vi "SelectData.vi"(8 "error in (no error)":errorcluster, 10 "Select Conditions Criteria":T1, 11 "object in":refnum<class "TableLogger_SQLite_Actor.lvclass">) -> (0 "error out":errorcluster, 2 "Data Clusters":variant[](array[variant]), 3 "object out":refnum<class "TableLogger_SQLite_Actor.lvclass">)   [LabVIEW 2014, in "TableLogger_SQLite_Actor.lvlib" / "TableLogger_SQLite_Actor.lvclass"]
uses:
  TableLogger_SQLite_Actor.lvclass
  TableLogger_Actor/SelectConditionCriteria.ctl
  SelectConditions.ctl
  TableLogger_SQLite_Actor.lvclass/TableLogger_SQLite_Actor.ctl
  <vilib>/drjdpowell/SQLite Library/SQL Connection/Execute SQL.vi
  <vilib>/drjdpowell/SQLite Library/SQLite.lvlib
  <vilib>/drjdpowell/SQLite Library/SQL Connection/Connection.lvclass
  TableLogger_Actor/TableLogger_Actor/TableLogger_Actor.lvclass
  TableLogger_Actor/TableLogger_Actor.lvlib
panel:
  # "Connector Pane"
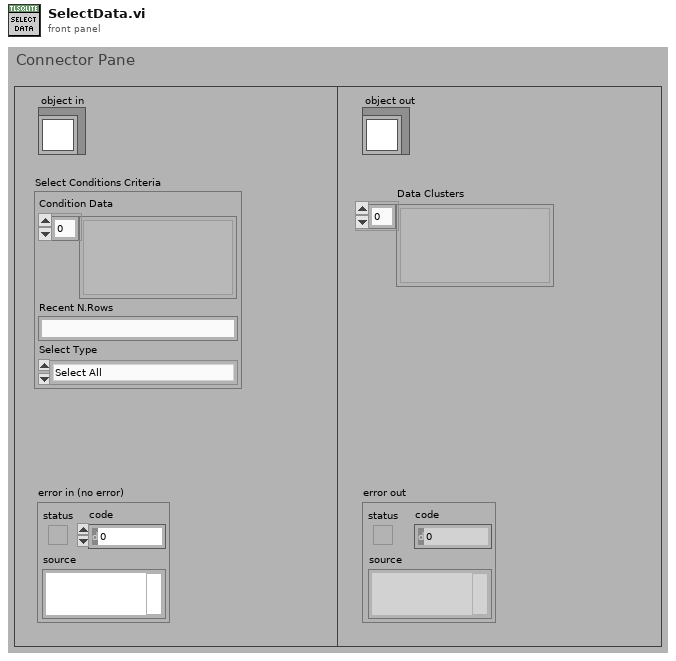
[diagram p1: front panel]
types:
  T1 = typedef "TableLogger_Actor.lvlib/SelectConditionCriteria.ctl" = cluster{"Condition Data":variant[], "Recent N.Rows":string, "Select Type":T2}
  T2 = typedef "TableLogger_Actor.lvlib/SelectConditions.ctl" = enum16{"Select All", "Select with AND Operator", "Select Most Recent Rows", "Select with OR Operator", "Select with BETWEEN Operator"}
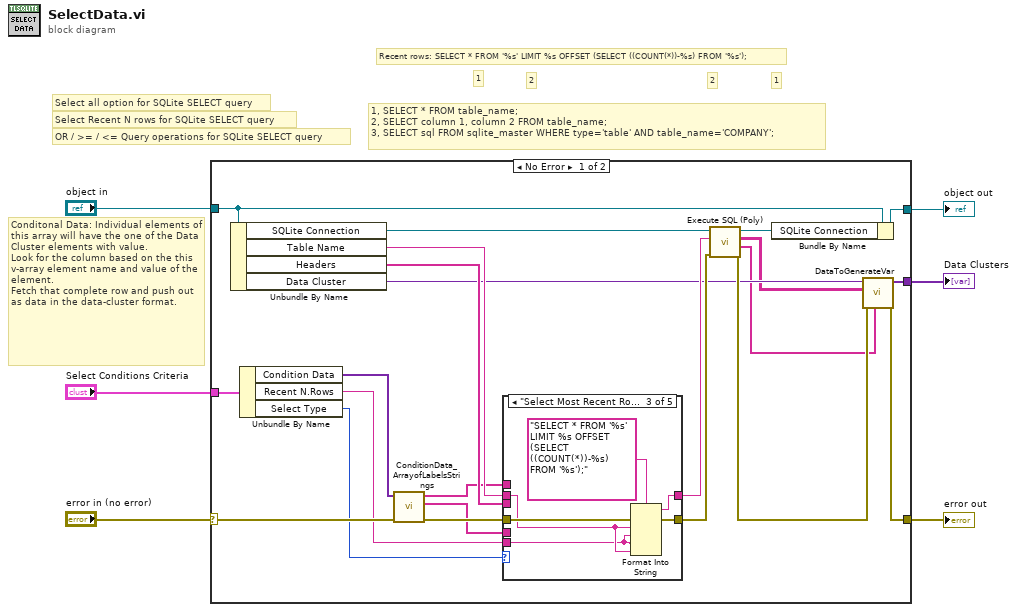
[diagram p0: block diagram]
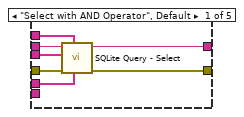
[diagram p2: hidden frame]
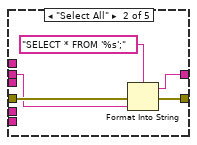
[diagram p3: hidden frame]
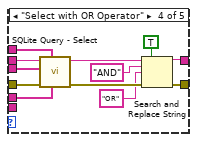
[diagram p4: hidden frame]
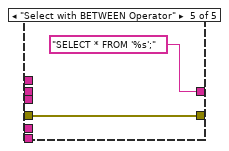
[diagram p5: hidden frame]
diagram:
  # "1"
  # "2"
  # "2"
  # "1"
  # "Recent rows: SELECT * FROM '%s' LIMIT %s OFFSET (SELECT ((COUNT(*))-%s) FROM '%s');"
  # "Select all option for SQLite SELECT query"
  # "Select Recent N rows for SQLite SELECT query"
  # "OR / >= / <= Query operations for SQLite SELECT query"
  # "1, SELECT * FROM table_name;\n2, SELECT column 1, column 2 FROM table_name;\n3, SELECT sql FROM sqlite_master WHERE type='table' AND table_name='COMPANY';"
  # "Conditonal Data: Individual elements of this array will have the one of the Data Cluster elements with value.\nLook for the column based on the this v-array element name and value of the element.\nFetch that complete row and push out as data in the data-cluster format."
  n1 = case shown="No Error" "error in (no error)" {
    selector: "error in (no error)" -> [w20 w62]
    tunnel: [w16 w62] -> w5
    tunnel: [w27 w61] -> w3
    tunnel: "object in" -> [w28 w61]
    tunnel: "Select Conditions Criteria" -> [w10 _]
    tunnel: [w18 _] -> w2
    frame No Error {
      n2 = Unbundle By Name(w28) -> ("SQLite Connection"=w26:refnum<class "Connection.lvclass">, "Table Name"=w24:string, "Headers"=w21:string[], "Data Cluster"=w15:variant)
      n3 = Unbundle By Name(w10) -> ("Condition Data"=w9:variant[], "Recent N.Rows"=w8:string, "Select Type"=w7:T2)
      n4 = call "ConditionData_ArrayofLabelsStrings.vi"("error in (no error)"=w20, "Condition Data"=w9) -> ("error out"=w19:errorcluster, "Value"=w11:string[], "Label"=w12:string[])  [unwired: 7 in]
      n5 = case shown="\"Select Most Recent Rows\"" w7 {
        tunnel: w24 -> [w35 w36 w42 w57 _]
        tunnel: [w34 w39 w45 w52 w60] -> w23
        tunnel: [w33 w38 w44 w49 "SELECT * FROM '%s';" ("SQL")] -> w22
        tunnel: w21 -> [w32 _ _ w56 _]
        tunnel: w19 -> [w31 w40 w46 w58 w60]
        tunnel: w12 -> [w30 _ _ w55 _]
        tunnel: w11 -> [w29 _ _ w54 _]
        tunnel: w8 -> [_ _ w41 _ _]
        frame "Select with AND Operator", Default {
          n6 = call "SQLite Query - Select.vi"("Column Value"=w29, "Columns Names"=w30, "error in"=w31, "Table Headers"=w32, "Table Name"=w35) -> ("error out"=w34:errorcluster, "SQLite Query"=w33:string)  [unwired: 5 in]
        }
        frame "Select All" {
          n7 = Format Into String(format string="SELECT * FROM '%s';" ("SQL"), error in=w40, w36) -> (resulting string=w38:string, error out=w39:errorcluster)  [unwired: 1 in]
        }
        frame "Select Most Recent Rows" {
          n8 = Format Into String(format string="SELECT * FROM '%s' LIMIT %s OFFSET (SELECT ((COUNT(*))-%s) FROM '%s');" ("SQL"), error in=w46, w42, w41, w41, w42) -> (resulting string=w44:string, error out=w45:errorcluster)  [unwired: 1 in]
        }
        frame "Select with OR Operator" {
          n9 = call "SQLite Query - Select.vi"("Column Value"=w54, "Columns Names"=w55, "error in"=w58, "Table Headers"=w56, "Table Name"=w57) -> ("error out"=w53:errorcluster, "SQLite Query"=w51:string)  [unwired: 5 in]
          n10 = Search and Replace String(replace all?=TRUE ("replace all? (F)"), input string=w51, search string="AND", replace string="OR" ("replace string (\"\")"), error in=w53) -> (result string=w49:string, error out=w52:errorcluster)  [unwired: 3 in, 2 out]
        }
        frame "Select with BETWEEN Operator" {
        }
      }
      n11 = call-poly <vilib>:"Execute SQL (Poly).vi"("error in (no error)"=w23, "SQL"=w22, "SQLite Connection in"=w26) -> ("error out"=w17:errorcluster, "Column Names"=w13:string[], "Result Set"=w14:string[][], "SQLite Connection"=w25:refnum<class "Connection.lvclass">)  [unwired: 5 in]
      n12 = Bundle By Name(cluster=w28, "SQLite Connection"=w25) -> (w27:refnum<class "TableLogger_SQLite_Actor.lvclass">)
      n13 = call "DataToGenerateVar.vi"("Header"=w13, "error in (no error)"=w17, "Data in"=w14, "Variant"=w15) -> ("error out"=w16:errorcluster, "Data"=w18:variant[])  [unwired: 6 in]
    }
    frame Error {
    }
  }
  "error out" <- w5
  "object out" <- w3
  "Data Clusters" <- w2
